vi "4. SJCubeRunExp.vi"() -> ()   [LabVIEW 2019, in "SJCube_ElvisIII.lvlib"]
uses:
  SJCube_ElvisIII.lvlib
  <vilib>/Platform/TimedLoop/XDataNode/XDataNode.xnode
  <vilib>/Platform/TimedLoop/XDataNode/timing_clust.ctl
  <vilib>/Platform/TimedLoop/XDataNode/XDNodeRunTimeDep.lvlib
  <vilib>/Platform/TimedLoop/XDataNode/wakeup.ctl
  <vilib>/Platform/TimedLoop/XDataNode/nitl_modes.ctl
  <vilib>/myRIO/Instrument Drivers/Utilities/Utilities.lvlib
  <vilib>/ptbypt/NI_PtbyPt.lvlib
  <vilib>/addons/control/pid/NI_PID_pid.lvlib
  <vilib>/addons/control/pid/pid.llb/PID (DBL).vi
  PendulumState.ctl
panel:
  in  "motorPID":T1={"proportional gain (Kc)"=7.0, "integral time (Ti, min)"=0.0, "derivative time (Td, min)"=0.0001}
  in  "PosPID":T1={"proportional gain (Kc)"=-0.05999999999999999, "integral time (Ti, min)"=0.05, "derivative time (Td, min)"=0.019999999999999997}
  in  "BalancePID":T1={"proportional gain (Kc)"=0.07999999999999999, "integral time (Ti, min)"=0.0, "derivative time (Td, min)"=0.0006}
  out "nowState":T2
  in  "NextState":T2
  in  "manual State":bool
  out "Waveform Chart":T3(graph)
  in  "Setpoint(deg)":dbl(knob) scale=80.0..-80.0
  out "error out":errorcluster
  out "Position(deg)":dbl(knob) scale=80.0..-80.0
  in  "Reset":bool
  in  "Stop Button":bool
  out "MotorResetPOS":dbl[](array[numeric])
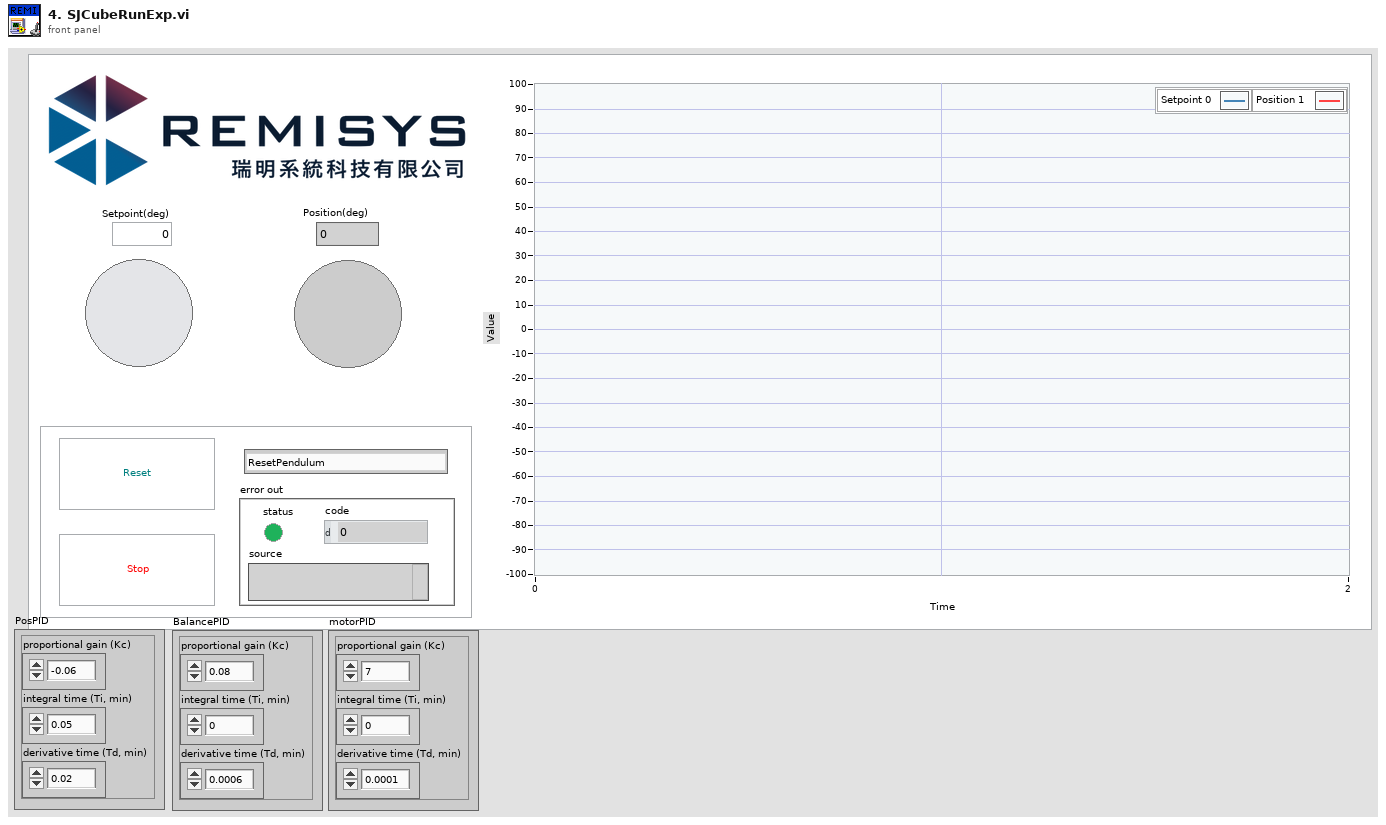
[diagram p1: front panel]
types:
  T1 = cluster{"proportional gain (Kc)":dbl, "integral time (Ti, min)":dbl, "derivative time (Td, min)":dbl}
  T2 = typedef "SJCube_ElvisIII.lvlib/PendulumState.ctl" = enum16{"ResetPendulum", "PendulumFindHome", "PendulumToHome", "SwingUp", "Balancing", "ExitExp."}
  T3 = cluster{"Setpoint(deg)":dbl, "PresentPOS(deg)":dbl}
  T4 = typedef "XDNodeRunTimeDep.lvlib/timing_clust.ctl" = cluster{"Expected End [f-1]":u64, "Actual End [f-1]":u64, "Finished Late? [f-1]":bool, "Expected End [i-1]":u64, "Actual End [i-1]":u64, "Finished Late? [i-1]":bool, "Expected Start [i]":u64, "Actual Start [i]":u64, "Expected Start [f]":u64, "Actual Start [f]":u64, "Source Name":string, "Structure Name":string, "Period":i64, "Deadline":i64, "Offset":i64, "Start":i64, "Priority":i32, "Timeout":i32, "Mode":T5, "Wakeup Reason":T6, "Error":errorcluster, "Source Type":string, "Secondary Source Type":string, "Global End Time":u64, "Global Start Time":u64, "Frame Duration":u64, "Iteration Duration":u64, "Assigned CPU":i32, "I/O Scan Engine Mode":u32}
  T5 = typedef "XDNodeRunTimeDep.lvlib/nitl_modes.ctl" = enum32{"No Change", "Process missed periods, maintain original phase", "Discard missed periods, maintain original phase", "Process missed periods, ignore original phase", "Discard missed periods, ignore original phase"}
  T6 = typedef "XDNodeRunTimeDep.lvlib/wakeup.ctl" = enum32{"Normal", "Aborted", "Asynchronous wakeup", "Timing source error", "Timed loop error", "Timeout"}
  T7 = cluster{"Setpoint(deg)":dbl, "MotorEncoder (deg)":dbl}
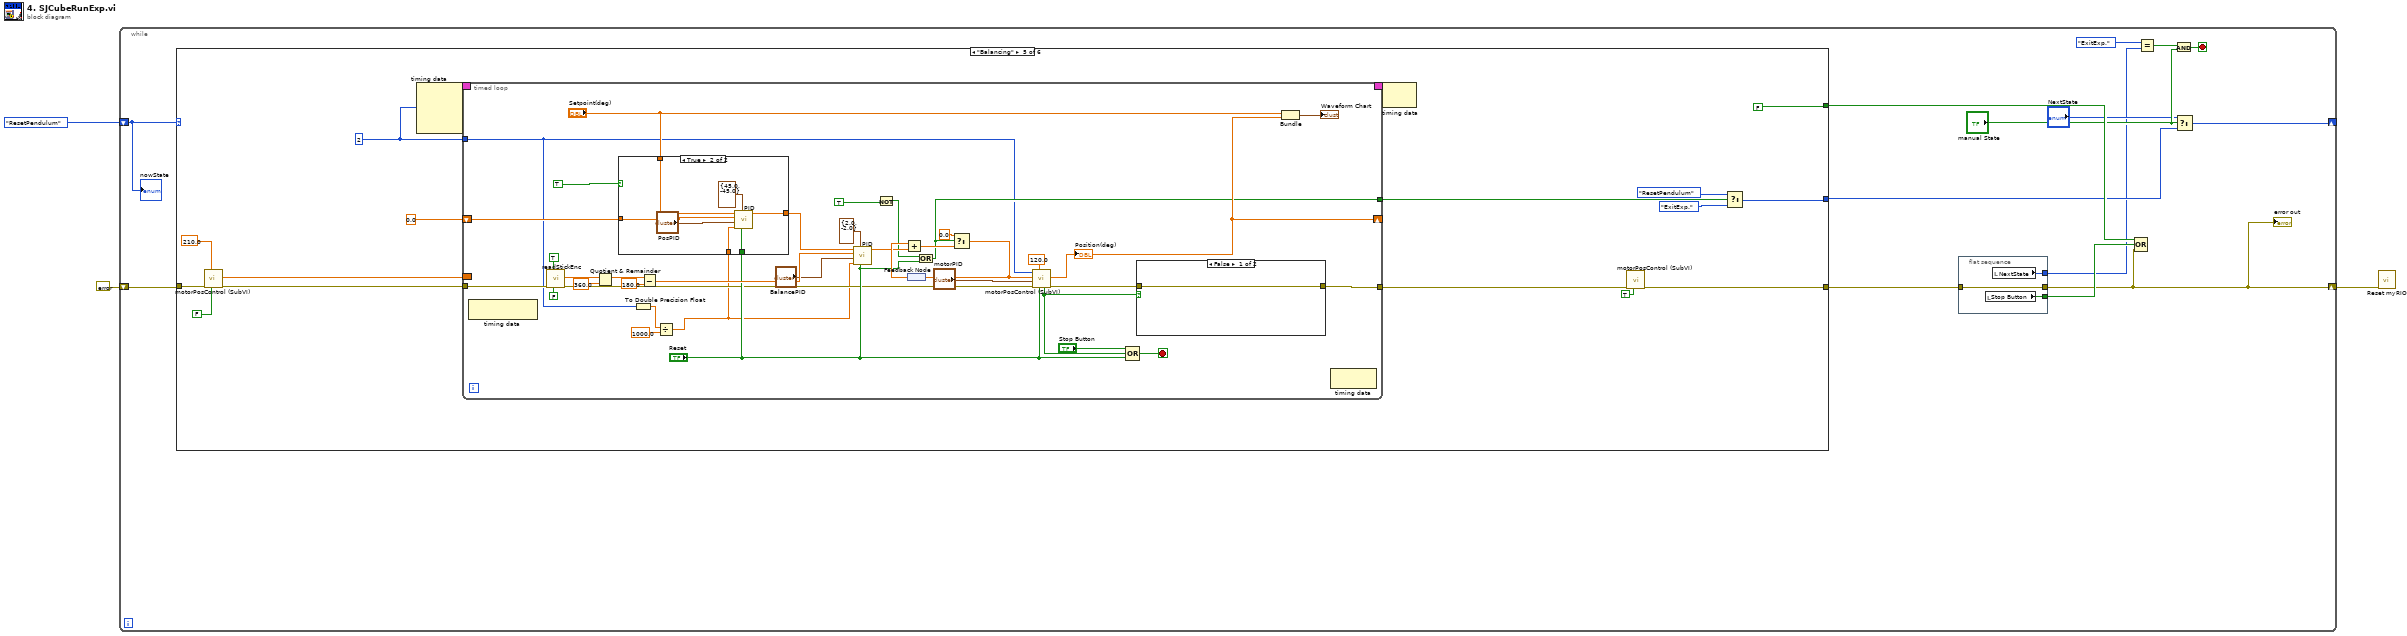
[diagram p0: block diagram]
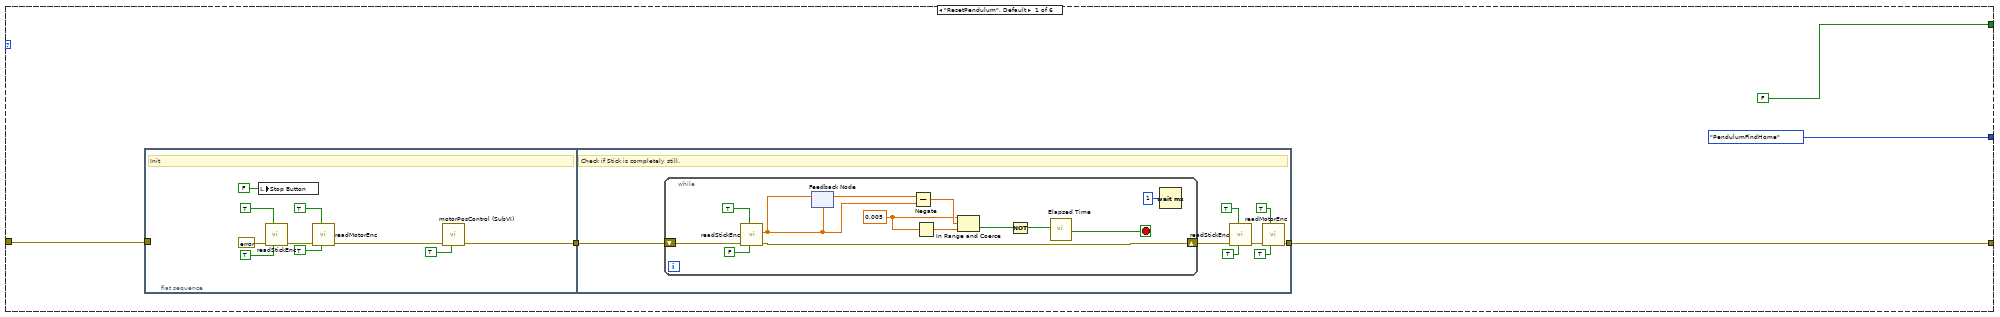
[diagram p2: hidden frame]
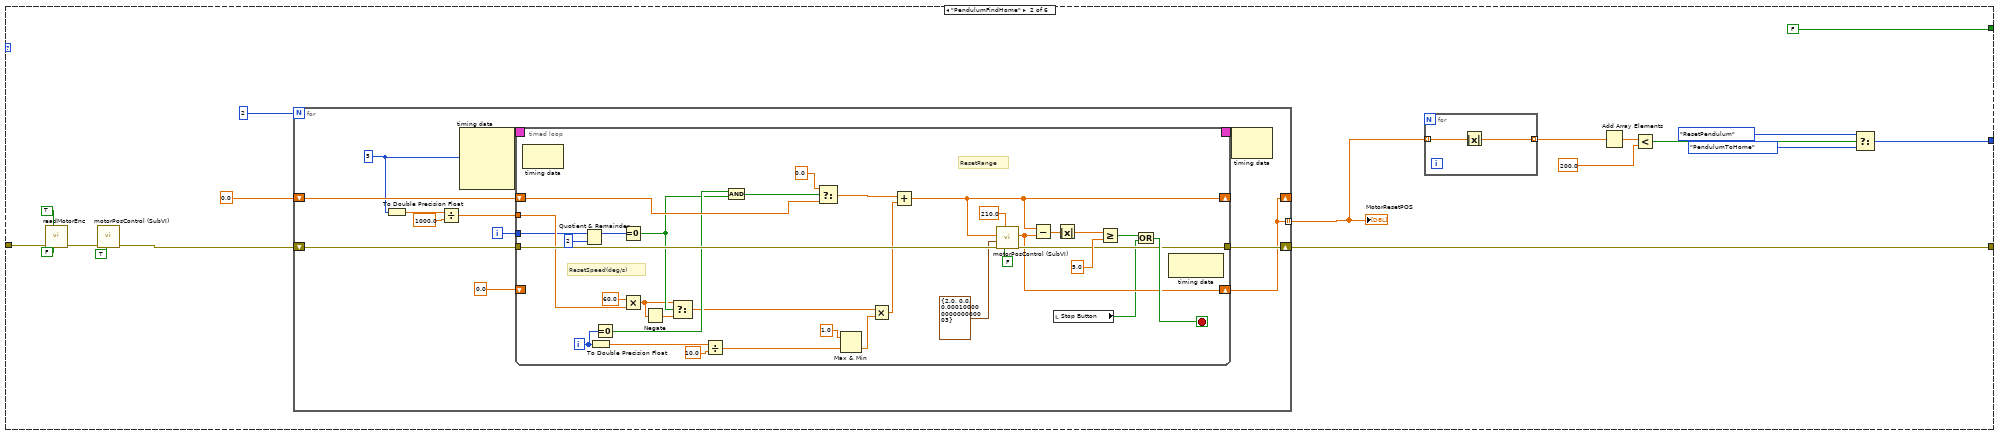
[diagram p3: hidden frame]
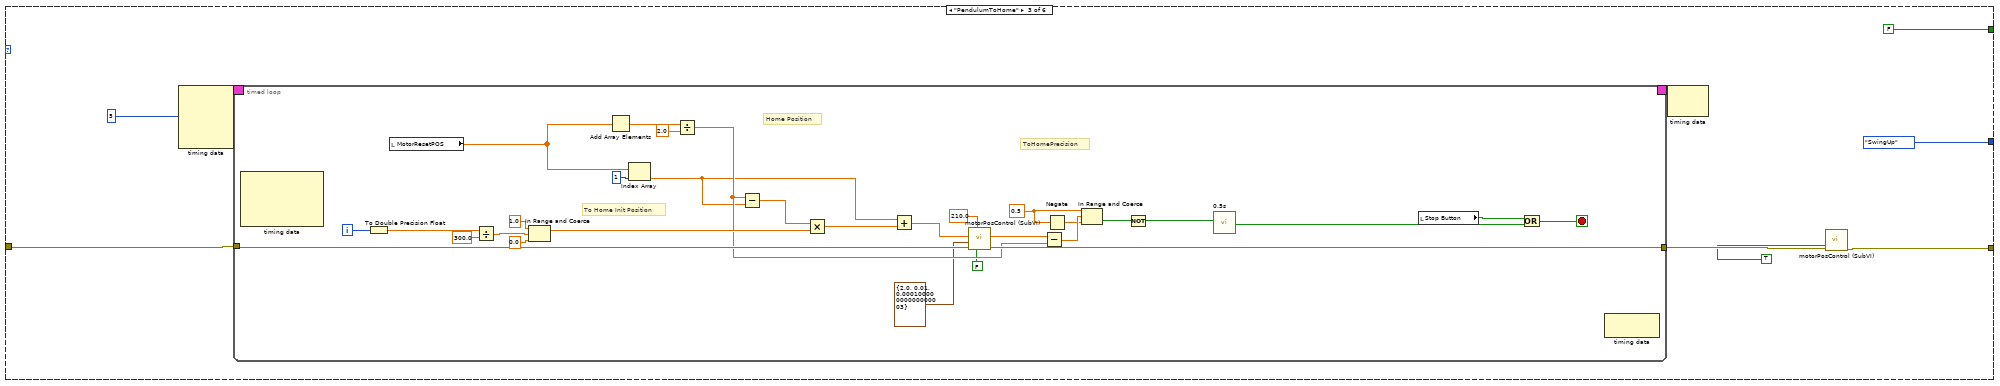
[diagram p4: hidden frame]
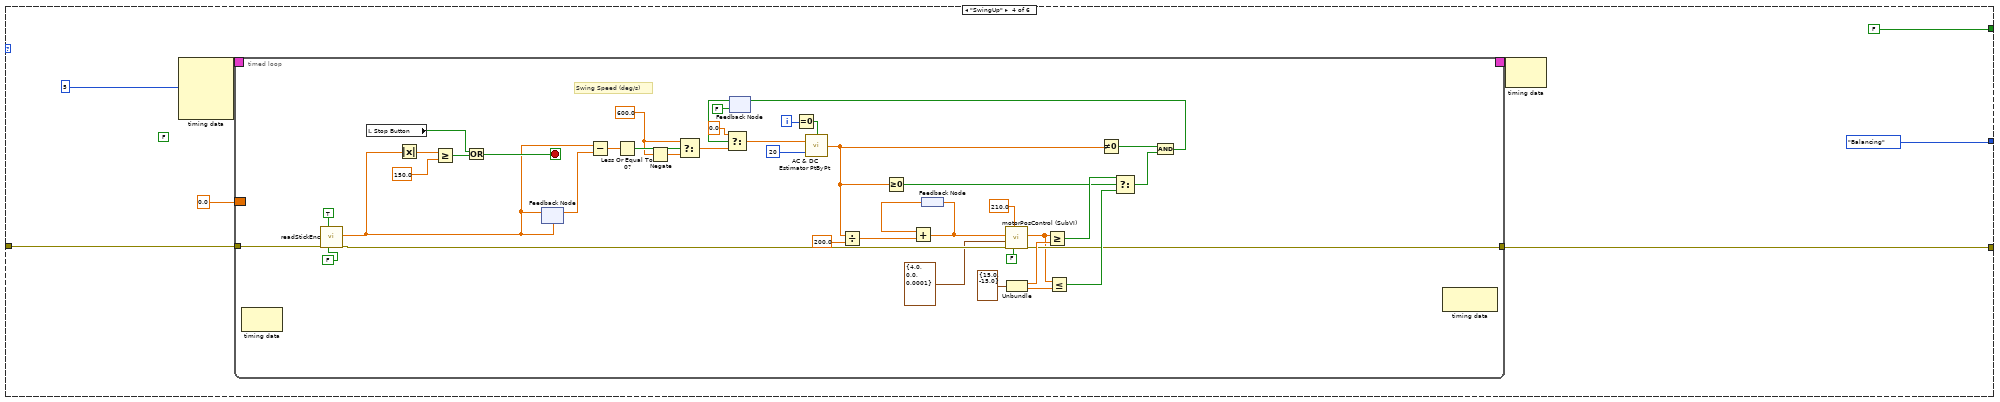
[diagram p5: hidden frame]
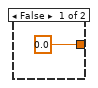
[diagram p6: hidden frame]
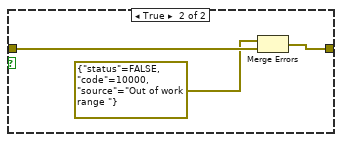
[diagram p7: hidden frame]
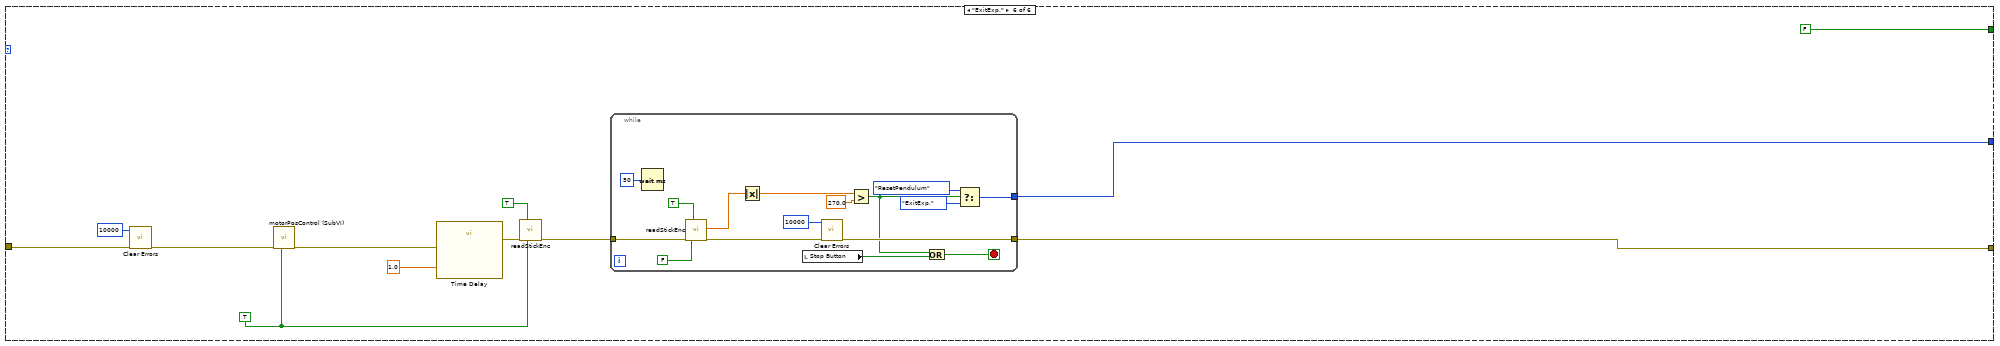
[diagram p8: hidden frame]
diagram:
  n1 = while {
    shift-right: [w11] -> _
    shift-left: PendulumState."ResetPendulum" ("Start State") -> [w13]
    shift-right: [w4] -> w1
    shift-left: errorcluster {"status"=FALSE, "code"=0, "source"=""} ("error in (no error)") -> [w17]
    stop <- w7 stop-if-true
    n2 = case shown="\"Balancing\"" w13 {
      tunnel: w17 -> [w23 w71 w134 w176 w246 w310]
      tunnel: [w24 w74 w130 w175 w243 w308] -> w16
      tunnel: [PendulumState."PendulumFindHome" w57 PendulumState."SwingUp" PendulumState."Balancing" w240 w312] -> w12
      tunnel: [FALSE FALSE FALSE FALSE FALSE FALSE] -> w14
      frame "ResetPendulum", Default {
        n3 = flat-sequence {
          tunnel: w23 -> [_]
          tunnel: [w27] -> w21
          tunnel: [w39] -> w24
          tunnel: w21 -> [w36]
          frame #0 {
            # "Init"
            n4 = local write "Stop Button"(FALSE ("Stop Button")) -> ()
            n5 = call "readStickEnc.vi"("Reset Counter"=TRUE, "Reverse ENC?"=TRUE, "error in (no error)"=errorcluster {"status"=FALSE, "code"=0, "source"=""}) -> ("error out"=w32:errorcluster)  [unwired: 7 in, 1 out]
            n6 = call "readMotorEnc.vi"("Reset Counter"=TRUE, "Reverse ENC?"=TRUE, "error in (no error)"=w32) -> ("error out"=w28:errorcluster)  [unwired: 7 in, 1 out]
            n7 = call "motorPosControl (SubVI).vi"("Reset"=TRUE, "error in (no error)"=w28) -> ("error out"=w27:errorcluster)  [unwired: 6 in, 3 out]
          }
          frame #1 {
            # "Check if Stick is completely still."
            n8 = while {
              shift-right: [w56] -> w43
              shift-left: w36 -> [w55]
              stop <- w46 stop-if-true
              w52 = 0.005 ("upper limit")
              n9 = call "readStickEnc.vi"("Reset Counter"=FALSE, "Reverse ENC?"=TRUE, "error in (no error)"=w55) -> ("error out"=w56:errorcluster, "StickEncoder (deg)"=w50:dbl)  [unwired: 7 in]
              n10 = feedback-in #1(w50) -> ()
              n11 = feedback #1(w50) -> (w54:dbl)
              n12 = Subtract(x=w54, y=w50) -> (x-y=w53:dbl)
              n13 = Negate(x=w52) -> (-x=w51:dbl)
              n14 = In Range and Coerce(upper limit=w52, x=w53, lower limit=w51) -> (In Range?=w48:bool)  [unwired: 1 out]
              n15 = Not(x=w48) -> (.not. x?=w47:bool)
              n16 = call "Elapsed Time"("Reset"=w47) -> ("Time has Elapsed"=w46:bool)  [unwired: 11 in, 7 out]
              n17 = Wait (ms)(milliseconds to wait=u32 1) -> ()  [unwired: 1 out]
            }
            n18 = call "readStickEnc.vi"("Reset Counter"=TRUE, "Reverse ENC?"=TRUE, "error in (no error)"=w43) -> ("error out"=w40:errorcluster)  [unwired: 7 in, 1 out]
            n19 = call "readMotorEnc.vi"("Reset Counter"=TRUE, "Reverse ENC?"=TRUE, "error in (no error)"=w40) -> ("error out"=w39:errorcluster)  [unwired: 7 in, 1 out]
          }
        }
      }
      frame "PendulumFindHome" {
        n20 = call "readMotorEnc.vi"("Reset Counter"=FALSE, "Reverse ENC?"=TRUE ("Reset Button"), "error in (no error)"=w71) -> ("error out"=w72:errorcluster)  [unwired: 7 in, 1 out]
        n21 = call "motorPosControl (SubVI).vi"("Reset"=TRUE, "error in (no error)"=w72) -> ("error out"=w66:errorcluster)  [unwired: 6 in, 3 out]
        n22 = for {
          N: 2 -> [_]
          shift-right: [w86] -> w74
          shift-left: w66 -> [w85]
          shift-right: [w78] -> _
          shift-left: 0.0 ("PresentPOS(deg)") -> [w83]
          tunnel: [w78] -> w64 mode=indexing
          i -> [w84]
          w82 = i64 5 ("Period")
          n23 = To Double Precision Float(number=w82) -> (double precision float=w81:dbl)
          n24 = Divide(x=w81, y=1000.0) -> (x/y=w79:dbl)
          n25 = node-c288(w82) -> (w88:T4)  [unwired: 3 in]
          n26 = timed-loop {
            timing: w88 -> [_]
            timing-out: [_] -> w87
            tunnel: w85 -> [w117]
            tunnel: [w116] -> w86
            tunnel: w84 -> [w100]
            shift-right: [w111] -> _
            shift-left: w83 -> [w99]
            tunnel: w79 -> [w107]
            shift-right: [w106] -> w78
            shift-left: 0.0 ("MotorEncoder (deg)") -> [_]
            i -> [w95]
            stop <- w121 stop-if-true
            # "ResetRange"
            # "ResetSpeed(deg/s)"
            n27 = node-c288() -> ()  [unwired: 1 in, 1 out]
            n28 = Quotient & Remainder(x=w100, y=2) -> (x-y*floor(x/y)=w96:i32)  [unwired: 1 out]
            n29 = To Double Precision Float(number=w95) -> (double precision float=w112:dbl)
            n30 = Equal To 0?(x=w95) -> (x = 0?=w93:bool)
            n31 = Equal To 0?(x=w96) -> (x = 0?=w92:bool)
            n32 = Multiply(x=60.0 ("y"), y=w107) -> (x*y=w91:dbl)
            n33 = Negate(x=w91) -> (-x=w90:dbl)
            n34 = Select(t=w91, s=w92, f=w90) -> (s? t:f=w89:dbl)
            n35 = Divide(x=w112, y=10.0) -> (x/y=w110:dbl)
            n36 = And(x=w93, y=w92) -> (x .and. y?=w94:bool)
            n37 = Select(t=0.0, s=w94, f=w99) -> (s? t:f=w97:dbl)
            n38 = Max & Min(x=1.0 ("upper limit"), y=w110) -> (min(x,y)=w105:dbl)  [unwired: 1 out]
            n39 = Multiply(x=w89, y=w105) -> (x*y=w102:dbl)
            n40 = Add(x=w97, y=w102) -> (x+y=w111:dbl)
            n41 = call "motorPosControl (SubVI).vi"("Reset"=FALSE, "+/- Range"=210.0 ("WorkRange"), "error in (no error)"=w117, "PID gains"=T1 {"proportional gain (Kc)"=2.0, "integral time (Ti, min)"=0.0, "derivative time (Td, min)"=0.00010000000000000003}, "Position (deg)"=w111) -> ("error out"=w116:errorcluster, "MotorEncoder (deg)"=w106:dbl)  [unwired: 3 in, 2 out]
            n42 = Subtract(x=w111, y=w106) -> (x-y=w119:dbl)
            n43 = local read "Stop Button"() -> (w103:bool)
            n44 = Absolute Value(x=w119) -> (abs(x)=w118:dbl)
            n45 = Greater Or Equal?(x=w118, y=5.0) -> (x >= y?=w104:bool)
            n46 = Or(x=w104, y=w103) -> (x .or. y?=w121:bool)
            n47 = node-c288() -> ()  [unwired: 1 in, 1 out]
          }
          n48 = node-c288(w87) -> ()  [unwired: 1 out]
        }
        "MotorResetPOS" <- w64
        n49 = for {
          tunnel: w64 -> [w76] mode=indexing
          tunnel: [w75] -> w63 mode=indexing
          n50 = Absolute Value(x=w76) -> (abs(x)=w75:dbl)
        }
        n51 = Add Array Elements(numeric array=w63) -> (sum=w62:dbl)
        n52 = Less?(x=w62, y=200.0) -> (x < y?=w60:bool)
        n53 = Select(t=PendulumState."ResetPendulum", s=w60, f=PendulumState."PendulumToHome") -> (s? t:f=w57:T2)
      }
      frame "PendulumToHome" {
        n54 = node-c288(i64 5 ("Period")) -> (w136:T4)  [unwired: 3 in]
        n55 = timed-loop {
          timing: w136 -> [_]
          timing-out: [_] -> w135
          tunnel: w134 -> [w167]
          tunnel: [w162] -> w132
          i -> [w161]
          stop <- w147 stop-if-true
          w164 = 0.5
          # "To Home Init Position"
          # "Home Position"
          # "ToHomePrecision"
          n56 = node-c288() -> ()  [unwired: 1 in, 4 out]
          n57 = To Double Precision Float(number=w161) -> (double precision float=w144:dbl)
          n58 = local read "MotorResetPOS"() -> (w156:dbl[])
          n59 = Divide(x=w144, y=300.0) -> (x/y=w159:dbl)
          n60 = In Range and Coerce(upper limit=1.0, x=w159, lower limit=0.0) -> (coerced(x)=w154:dbl)  [unwired: 1 out]
          n61 = Add Array Elements(numeric array=w156) -> (sum=w155:dbl)
          n62 = Index Array(array=w156, index=1) -> (element=w150:dbl)
          n63 = Divide(x=w155, y=2.0) -> (x/y=w152:dbl)
          n64 = Subtract(x=w152, y=w150) -> (x-y=w151:dbl)
          n65 = Multiply(x=w151, y=w154) -> (x*y=w153:dbl)
          n66 = Add(x=w150, y=w153) -> (x+y=w149:dbl)
          n67 = call "motorPosControl (SubVI).vi"("Reset"=FALSE, "+/- Range"=210.0 ("WorkRange"), "error in (no error)"=w167, "PID gains"=T1 {"proportional gain (Kc)"=2.0, "integral time (Ti, min)"=0.01, "derivative time (Td, min)"=0.00010000000000000003}, "Position (deg)"=w149) -> ("error out"=w162:errorcluster, "MotorEncoder (deg)"=w166:dbl)  [unwired: 3 in, 2 out]
          n68 = Subtract(x=w166, y=w152) -> (x-y=w165:dbl)
          n69 = Negate(x=w164) -> (-x=w163:dbl)
          n70 = In Range and Coerce(upper limit=w164, x=w165, lower limit=w163) -> (In Range?=w142:bool)  [unwired: 1 out]
          n71 = Not(x=w142) -> (.not. x?=w141:bool)
          n72 = call "0.5s"("Reset"=w141) -> ("Time has Elapsed"=w139:bool)  [unwired: 11 in, 7 out]
          n73 = local read "Stop Button"() -> (w138:bool)
          n74 = Or(x=w138, y=w139) -> (x .or. y?=w147:bool)
          n75 = node-c288() -> ()  [unwired: 1 in, 1 out]
        }
        n76 = node-c288(w135) -> ()  [unwired: 1 out]
        n77 = call "motorPosControl (SubVI).vi"("Reset"=TRUE ("Reset Button"), "error in (no error)"=w132) -> ("error out"=w130:errorcluster)  [unwired: 6 in, 3 out]
      }
      frame "SwingUp" {
        (unwired) FALSE
        n78 = node-c288(i64 5 ("Period")) -> (w179:T4)  [unwired: 3 in]
        n79 = timed-loop {
          timing: w179 -> [_]
          timing-out: [_] -> w178
          tunnel: w176 -> [w201]
          tunnel: [w200] -> w175
          border: 0.0 -> [_]
          i -> [w223]
          stop <- w219 stop-if-true
          w215 = 600.0 ("MaxSpeed(deg/s)")
          # "Swing Speed (deg/s)"
          n80 = node-c288() -> ()  [unwired: 1 in, 1 out]
          n81 = call "readStickEnc.vi"("Reset Counter"=FALSE, "Reverse ENC?"=TRUE, "error in (no error)"=w201) -> ("error out"=w198:errorcluster, "StickEncoder (deg)"=w192:dbl)  [unwired: 7 in]
          n82 = local read "Stop Button"() -> (w196:bool)
          n83 = Absolute Value(x=w192) -> (abs(x)=w221:dbl)
          n84 = Greater Or Equal?(x=w221, y=150.0) -> (x >= y?=w197:bool)
          n85 = Or(x=w196, y=w197) -> (x .or. y?=w219:bool)
          n86 = feedback-in #2(w192) -> ()
          n87 = feedback #2(w192) -> (w222:dbl)
          n88 = Subtract(x=w192, y=w222) -> (x-y=w218:dbl)
          n89 = Less Or Equal To 0?(x=w218) -> (x <= 0?=w217:bool)
          n90 = Negate(x=w215) -> (-x=w216:dbl)
          n91 = Select(t=w215, s=w217, f=w216) -> (s? t:f=w211:dbl)
          n92 = feedback #3(FALSE) -> (w212:bool)
          n93 = Select(t=0.0, s=w212, f=w211) -> (s? t:f=w191:dbl)
          n94 = Equal To 0?(x=w223) -> (x = 0?=w185:bool)
          n95 = call <vilib>:"AC & DC Estimator PtByPt.vi"("signal"=w191, "sample length"=20, "initialize"=w185) -> ("DC estimate (V)"=w190:dbl)  [unwired: 2 out]
          n96 = Divide(x=w190, y=200.0 ("x")) -> (x/y=w189:dbl)
          n97 = Greater Or Equal To 0?(x=w190) -> (x >= 0?=w195:bool)
          n98 = feedback #4() -> (w214:dbl)
          n99 = Add(x=w214, y=w189) -> (x+y=w188:dbl)
          n100 = feedback-in #4(w188) -> ()
          n101 = call "motorPosControl (SubVI).vi"("Reset"=FALSE, "+/- Range"=210.0 ("WorkRange"), "error in (no error)"=w198, "PID gains"=T1 {"proportional gain (Kc)"=4.0, "integral time (Ti, min)"=0.0, "derivative time (Td, min)"=0.0001}, "Position (deg)"=w188) -> ("error out"=w200:errorcluster, "MotorEncoder (deg)"=w193:dbl)  [unwired: 3 in, 2 out]
          n102 = Unbundle(cluster{"UpLimit":dbl, "DownLimit":dbl} {"UpLimit"=15.0, "DownLimit"=-15.0} ("RunUpLimuit")) -> ("UpLimit"=w208:dbl, "DownLimit"=w207:dbl)
          n103 = Greater Or Equal?(x=w193, y=w208) -> (x >= y?=w206:bool)
          n104 = Less Or Equal?(x=w193, y=w207) -> (x <= y?=w205:bool)
          n105 = Not Equal To 0?(x=w190) -> (x != 0?=w204:bool)
          n106 = Select(t=w206, s=w195, f=w205) -> (s? t:f=w203:bool)
          n107 = And(x=w204, y=w203) -> (x .and. y?=w194:bool)
          n108 = feedback-in #3(w194) -> ()
          n109 = node-c288() -> ()  [unwired: 1 in, 1 out]
        }
        n110 = node-c288(w178) -> ()  [unwired: 1 out]
      }
      frame "Balancing" {
        w230 = i64 2 ("Period")
        n111 = call "motorPosControl (SubVI).vi"("Reset"=FALSE ("Reset Button"), "+/- Range"=210.0, "error in (no error)"=w246) -> ("error out"=w235:errorcluster, "MotorEncoder (deg)"=w234:dbl)  [unwired: 5 in, 2 out]
        n112 = node-c288(w230) -> (w238:T4)  [unwired: 3 in]
        n113 = timed-loop "Timed Loop" {
          timing: w238 -> [_]
          timing-out: [_] -> w237
          border: w234 -> [_]
          shift-right: [w255] -> _
          shift-left: 0.0 -> [w256]
          tunnel: w235 -> [w263]
          tunnel: [w253] -> w233
          tunnel: [w261] -> w232
          tunnel: w230 -> [w247]
          stop <- w273 stop-if-true
          n114 = node-c288() -> ()  [unwired: 1 in, 1 out]
          n115 = call "readStickEnc.vi"("Reset Counter"=FALSE, "Reverse ENC?"=TRUE, "error in (no error)"=w263) -> ("error out"=w265:errorcluster, "StickEncoder (deg)"=w266:dbl)  [unwired: 7 in]
          n116 = Quotient & Remainder(x=w266, y=360.0) -> (x-y*floor(x/y)=w274:dbl)  [unwired: 1 out]
          n117 = To Double Precision Float(number=w247) -> (double precision float=w248:dbl)
          n118 = Subtract(x=w274, y=180.0) -> (x-y=w279:dbl)
          n119 = Divide(x=w248, y=1000.0) -> (x/y=w249:dbl)
          n120 = case shown="True" TRUE ("StickPosControl") {
            tunnel: w249 -> [_ w291]
            tunnel: [0.0 ("output") w289] -> w276
            tunnel: w256 -> [_ w288]
            tunnel: "Reset" -> [_ w287]
            tunnel: "Setpoint(deg)" -> [_ w285]
            frame False {
            }
            frame True {
              n121 = call-poly <vilib>:"PID.vi"("reinitialize? (F)"=w287, "output range"=cluster{"output high":dbl, "output low":dbl} {"output high"=45.0, "output low"=-45.0}, "dt (s)"=w291, "PID gains"="PosPID", "process variable"=w288, "setpoint"=w285) -> ("output"=w289:dbl)  [unwired: 4 in, 1 out]
            }
          }
          n122 = call-poly <vilib>:"PID.vi"("reinitialize? (F)"="Reset", "output range"=cluster{"output high":dbl, "output low":dbl} {"output high"=2.0, "output low"=-2.0}, "dt (s)"=w249, "PID gains"="BalancePID", "process variable"=w279, "setpoint"=w276) -> ("output"=w277:dbl)  [unwired: 4 in, 1 out]
          n123 = Not(x=TRUE ("BalanceControl")) -> (.not. x?=w251:bool)
          n124 = feedback #5() -> (w282:dbl)
          n125 = Add(x=w282, y=w277) -> (x+y=w281:dbl)
          n126 = Or(x=w251, y="Reset") -> (x .or. y?=w253:bool)
          n127 = Select(t=0.0, s=w253, f=w281) -> (s? t:f=w268:dbl)
          n128 = feedback-in #5(w268) -> ()
          n129 = call "motorPosControl (SubVI).vi"("Reset"="Reset", "+/- Range"=120.0 ("WorkRange"), "error in (no error)"=w265, "PID gains"="motorPID", "Position (deg)"=w268, "dt"=w247) -> ("error out"=w270:errorcluster, "MotorEncoder (deg)"=w255:dbl, "out of range!"=w271:bool)  [unwired: 2 in, 1 out]
          "Position(deg)" <- w255
          n130 = Compound Arithmetic op=OR("Stop Button", w271, "Reset") -> (w273:bool)
          n131 = case shown="False" w271 {
            tunnel: w270 -> [w292 w295]
            tunnel: [w292 w294] -> w261
            frame False {
            }
            frame True {
              n132 = Merge Errors(errorcluster {"status"=FALSE, "code"=10000, "source"="Out of work range "} ("error in (no error)"), w295) -> (w294:errorcluster)
            }
          }
          n133 = Bundle("Setpoint(deg)"="Setpoint(deg)", "MotorEncoder (deg)"=w255) -> (→"Waveform Chart":T7)  [unwired: 1 in]
          n134 = node-c288() -> ()  [unwired: 1 in, 1 out]
        }
        n135 = node-c288(w237) -> ()  [unwired: 1 out]
        n136 = call "motorPosControl (SubVI).vi"("Reset"=TRUE ("Reset Button"), "error in (no error)"=w232) -> ("error out"=w243:errorcluster)  [unwired: 6 in, 3 out]
        n137 = Select(t=PendulumState."ResetPendulum", s=w233, f=PendulumState."ExitExp.") -> (s? t:f=w240:T2)
      }
      frame "ExitExp." {
        w305 = TRUE ("Reset Counter")
        n138 = call <vilib>:"Clear Errors.vi"("error in (no error)"=w310, "specific error code to clear (0: all)"=10000) -> ("error out"=w307:errorcluster)  [unwired: 4 in, 1 out]
        n139 = call "motorPosControl (SubVI).vi"("Reset"=w305, "error in (no error)"=w307) -> ("error out"=w306:errorcluster)  [unwired: 6 in, 3 out]
        n140 = call "Time Delay"("error in (no error)"=w306, "Delay Time (s)"=1.0) -> ("error out"=w304:errorcluster)  [unwired: 9 in]
        n141 = call "readStickEnc.vi"("Reset Counter"=w305, "Reverse ENC?"=TRUE, "error in (no error)"=w304) -> ("error out"=w303:errorcluster)  [unwired: 7 in, 1 out]
        n142 = while {
          tunnel: w303 -> [w329]
          tunnel: [w323] -> w312
          tunnel: [w319] -> w308
          stop <- w316 stop-if-true
          n143 = Wait (ms)(milliseconds to wait=u32 50) -> ()  [unwired: 1 out]
          n144 = call "readStickEnc.vi"("Reset Counter"=FALSE, "Reverse ENC?"=TRUE, "error in (no error)"=w329) -> ("error out"=w320:errorcluster, "StickEncoder (deg)"=w326:dbl)  [unwired: 7 in]
          n145 = Absolute Value(x=w326) -> (abs(x)=w318:dbl)
          n146 = local read "Stop Button"() -> (w315:bool)
          n147 = call <vilib>:"Clear Errors.vi"("error in (no error)"=w320, "specific error code to clear (0: all)"=10000) -> ("error out"=w319:errorcluster)  [unwired: 4 in, 1 out]
          n148 = Greater?(x=w318, y=270.0) -> (0:w314:bool)
          n149 = Or(x=w314, y=w315) -> (x .or. y?=w316:bool)
          n150 = Select(t=PendulumState."ResetPendulum", s=w314, f=PendulumState."ExitExp.") -> (s? t:f=w323:T2)
        }
      }
    }
    n151 = flat-sequence {
      tunnel: w16 -> [w19]
      tunnel: [w20] -> w15
      tunnel: [w19] -> w4
      tunnel: [w18] -> w5
      frame #0 {
        n152 = local read "Stop Button"() -> (w20:bool)
        n153 = local read "NextState"() -> (w18:T2)
      }
    }
    n154 = Compound Arithmetic op=OR(w14, w15, w4) -> ()  [unwired: 1 out]
    n155 = Equal?(x=PendulumState."ExitExp." ("y"), y=w5) -> (x = y?=w8:bool)
    n156 = And(x=w8, y="manual State") -> (x .and. y?=w7:bool)
    n157 = Select(t="NextState", s="manual State", f=w12) -> (s? t:f=w11:T2)
    "error out" <- w4
    "nowState" <- w13
  }
  n158 = call <vilib>:"Reset myRIO.vi"("error in (no error)"=w1) -> ()  [unwired: 10 in, 1 out]
